vi "List.vi"(8 "error in (no error)":errorcluster, 11 "LUnit Test Case In":refnum<class "LUnit Test Case.lvclass">) -> (0 "error out":errorcluster, 2 "List of Runnables":string[](array[string]))   [LabVIEW 2020]
uses:
  LUnit Test Case.lvclass
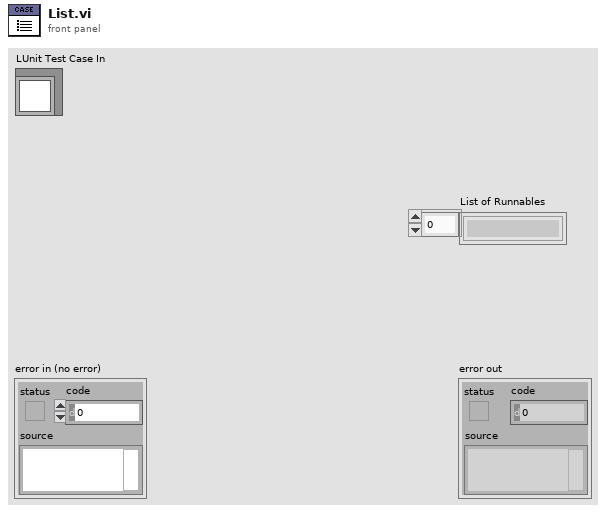
[diagram p1: front panel]
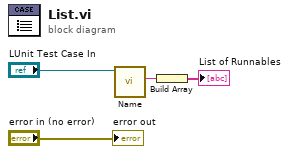
[diagram p0: block diagram]
diagram:
  n1 = call-dynamic "Name.vi"("LUnit Test Case in"="LUnit Test Case In") -> ("Name"=w1:string)  [unwired: 8 in, 2 out]
  n2 = Build Array(w1) -> (→"List of Runnables":string[])
  "error out" <- "error in (no error)"
